vi "Edit User.vi"(0 "User Manager View in":refnum<class "User Manager View.lvclass">, 5 "OldVal":T1, 11 "error in (no error)":errorcluster) -> (4 "User Manager View out":refnum<class "User Manager View.lvclass">, 15 "error out":errorcluster)   [LabVIEW 2017, in "User Manager View.lvlib" / "User Manager View.lvclass"]
uses:
  <vilib>/gpm_packages/@cs/User Manager App/User Manager View/User Manager View/User Manager View.lvclass
  <vilib>/gpm_packages/@cs/User Manager App/User Manager View/User Manager View/User Manager View.lvclass/User Manager View.ctl
  <vilib>/gpm_packages/@cs/User Manager App/User Manager View/User Manager Type Defs/State.ctl
  <vilib>/gpm_packages/@cs/User Manager App/User Manager View/User Manager View.lvlib
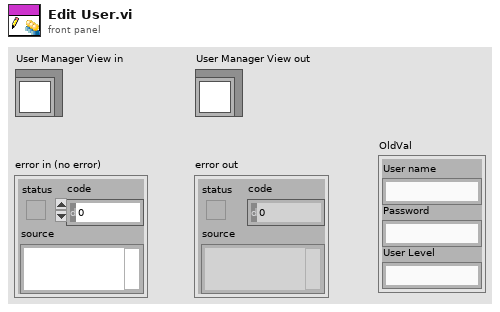
[diagram p1: front panel]
types:
  T1 = cluster{"User name":string, "Password":string, "User Level":string}
  T2 = enum8{"Enabled", "Disabled", "Disabled and Grayed Out"}
  T3 = typedef "User Manager View.lvlib/State.ctl" = enum16{"Normal", "Adding User", "Changing User Data"}
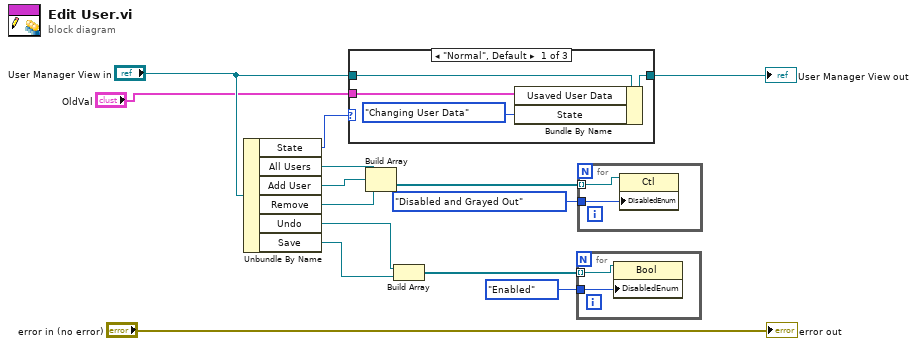
[diagram p0: block diagram]
diagram:
  n1 = Unbundle By Name("User Manager View in") -> ("State"=w1:T3, "All Users"=w10:refnum<vi>, "Add User"=w9:refnum<vi>, "Remove"=w4:refnum<vi>, "Undo"=w3:refnum<vi>, "Save"=w2:refnum<vi>)
  n2 = case shown="\"Normal\", Default" w1 {
    tunnel: "User Manager View in" -> [w18 w19 w20]
    tunnel: [w17 w19 w20] -> w12
    tunnel: "OldVal" -> [w16 _ _]
    frame "Normal", Default {
      n3 = Bundle By Name(cluster=w18, "Usaved User Data"=w16, "State"=State."Changing User Data") -> (w17:refnum<class "User Manager View.lvclass">)
    }
    frame "Changing User Data" {
    }
    frame "Adding User" {
    }
  }
  "User Manager View out" <- w12
  n4 = Build Array(w10, w9, w4) -> (w8:refnum<vi>[])
  n5 = Build Array(w3, w2) -> (w5:refnum<vi>[])
  n6 = for {
    tunnel: w5 -> [w22] mode=indexing
    tunnel: T2."Enabled" ("Disabled") -> [w21]
    n7 = property class="Bool"(reference=w22, "DisabledEnum"=w21) -> ()  [unwired: 1 in, 2 out]
  }
  n8 = for {
    tunnel: w8 -> [w24] mode=indexing
    tunnel: T2."Disabled and Grayed Out" ("Disabled") -> [w23]
    n9 = property class="Ctl"(reference=w24, "DisabledEnum"=w23) -> ()  [unwired: 1 in, 2 out]
  }
  "error out" <- "error in (no error)"
